vi "DataLogging_timing_test.vi"() -> ()   [LabVIEW 2018]
uses:
  Target Logging Cluster.ctl
  Logging Data Cluster.ctl
  Target Logging Control Signals.ctl
  Target Logging Sensors.ctl
  Sensor Data.ctl
  <vilib>/Platform/TimedLoop/XDataNode/timing_clust.ctl
  <vilib>/Platform/TimedLoop/XDataNode/nitl_modes.ctl
  <vilib>/Platform/TimedLoop/XDataNode/wakeup.ctl
  <vilib>/Analysis/baseanly.llb/Mean (DBL).vi
  <vilib>/platform/TimedLoop/XDataNode/XDataNode.xnode
  <vilib>/Platform/TimedLoop/XDataNode/XDNodeRunTimeDep.lvlib
  <vilib>/Analysis/NI_AALBase.lvlib
panel:
  out "mean (microseconds)":dbl format="%0.2f"
  out "Loop Duration Chart":i64(graph)
  in  "stop":bool
  out "Elapsed Time (ms)":u32
  out "Data Logging Error":errorcluster
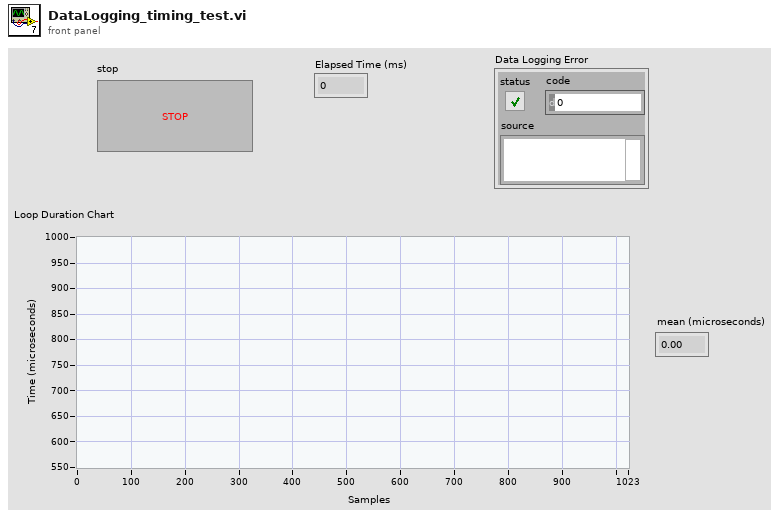
[diagram p1: front panel]
types:
  T1 = typedef "Target Logging Cluster.ctl" = cluster{"Valid for Logging?":bool, "Data":T2}
  T2 = typedef "Logging Data Cluster.ctl" = cluster{"Control Signals":T3, "Target Sensors":T4}
  T3 = typedef "Target Logging Control Signals.ctl" = cluster{"Phi":dbl, "Gait %":dbl, "ILC Desired Ankle Angle":dbl, "Desired Motor Current":dbl, "Transmission Ratio":dbl, "Passive Torque Estimate":dbl, "Torque Reference":dbl, "Left HS?":bool, "Left HS State":u32, "Right HS?":bool, "Right HS State":u32, "dGRF L":dbl, "dGRF R":dbl, "GRF L (filt) ":dbl, "GRF R (filt)":dbl}
  T4 = typedef "Target Logging Sensors.ctl" = cluster{"Sensors":T5}
  T5 = typedef "Sensor Data.ctl" = cluster{"Motor Current":dbl, "Motor Velocity":dbl, "Ankle Encoder Angle":dbl, "GRF L":dbl, "GRF R":dbl, "Index pulse?":bool, "Roll":dbl, "Pitch":dbl, "Yaw":dbl, "Thigh Angle":dbl}
  T6 = typedef "XDNodeRunTimeDep.lvlib/timing_clust.ctl" = cluster{"Expected End [f-1]":u64, "Actual End [f-1]":u64, "Finished Late? [f-1]":bool, "Expected End [i-1]":u64, "Actual End [i-1]":u64, "Finished Late? [i-1]":bool, "Expected Start [i]":u64, "Actual Start [i]":u64, "Expected Start [f]":u64, "Actual Start [f]":u64, "Source Name":string, "Structure Name":string, "Period":i64, "Deadline":i64, "Offset":i64, "Start":i64, "Priority":i32, "Timeout":i32, "Mode":T7, "Wakeup Reason":T8, "Error":errorcluster, "Source Type":string, "Secondary Source Type":string, "Global End Time":u64, "Global Start Time":u64, "Frame Duration":u64, "Iteration Duration":u64, "Assigned CPU":i32, "I/O Scan Engine Mode":u32}
  T7 = typedef "XDNodeRunTimeDep.lvlib/nitl_modes.ctl" = enum32{"No Change", "Process missed periods, maintain original phase", "Discard missed periods, maintain original phase", "Process missed periods, ignore original phase", "Discard missed periods, ignore original phase"}
  T8 = typedef "XDNodeRunTimeDep.lvlib/wakeup.ctl" = enum32{"Normal", "Aborted", "Asynchronous wakeup", "Timing source error", "Timed loop error", "Timeout"}
  T9 = typedef "Target Lossy Data.ctl" = cluster{"Active Controller":bool, "Log Trigger":bool, "Sensors":T5, "Motor Command":dbl, "Phase Variable":dbl, "Left HS State":u32, "Left Heel Strike Pulse":bool, "Gait %":dbl, "Torque Reference":dbl, "Passive Torque":dbl, "F_th":dbl, "dF_th":dbl, "d_GRF L":dbl, "GRF L":dbl, "Transmission Ratio":dbl, "Desired Ankle Traj.":dbl, "Right HS State":u32, "Right Heel Strike Pulse":bool, "d_GRF R":dbl, "GRF R":dbl}
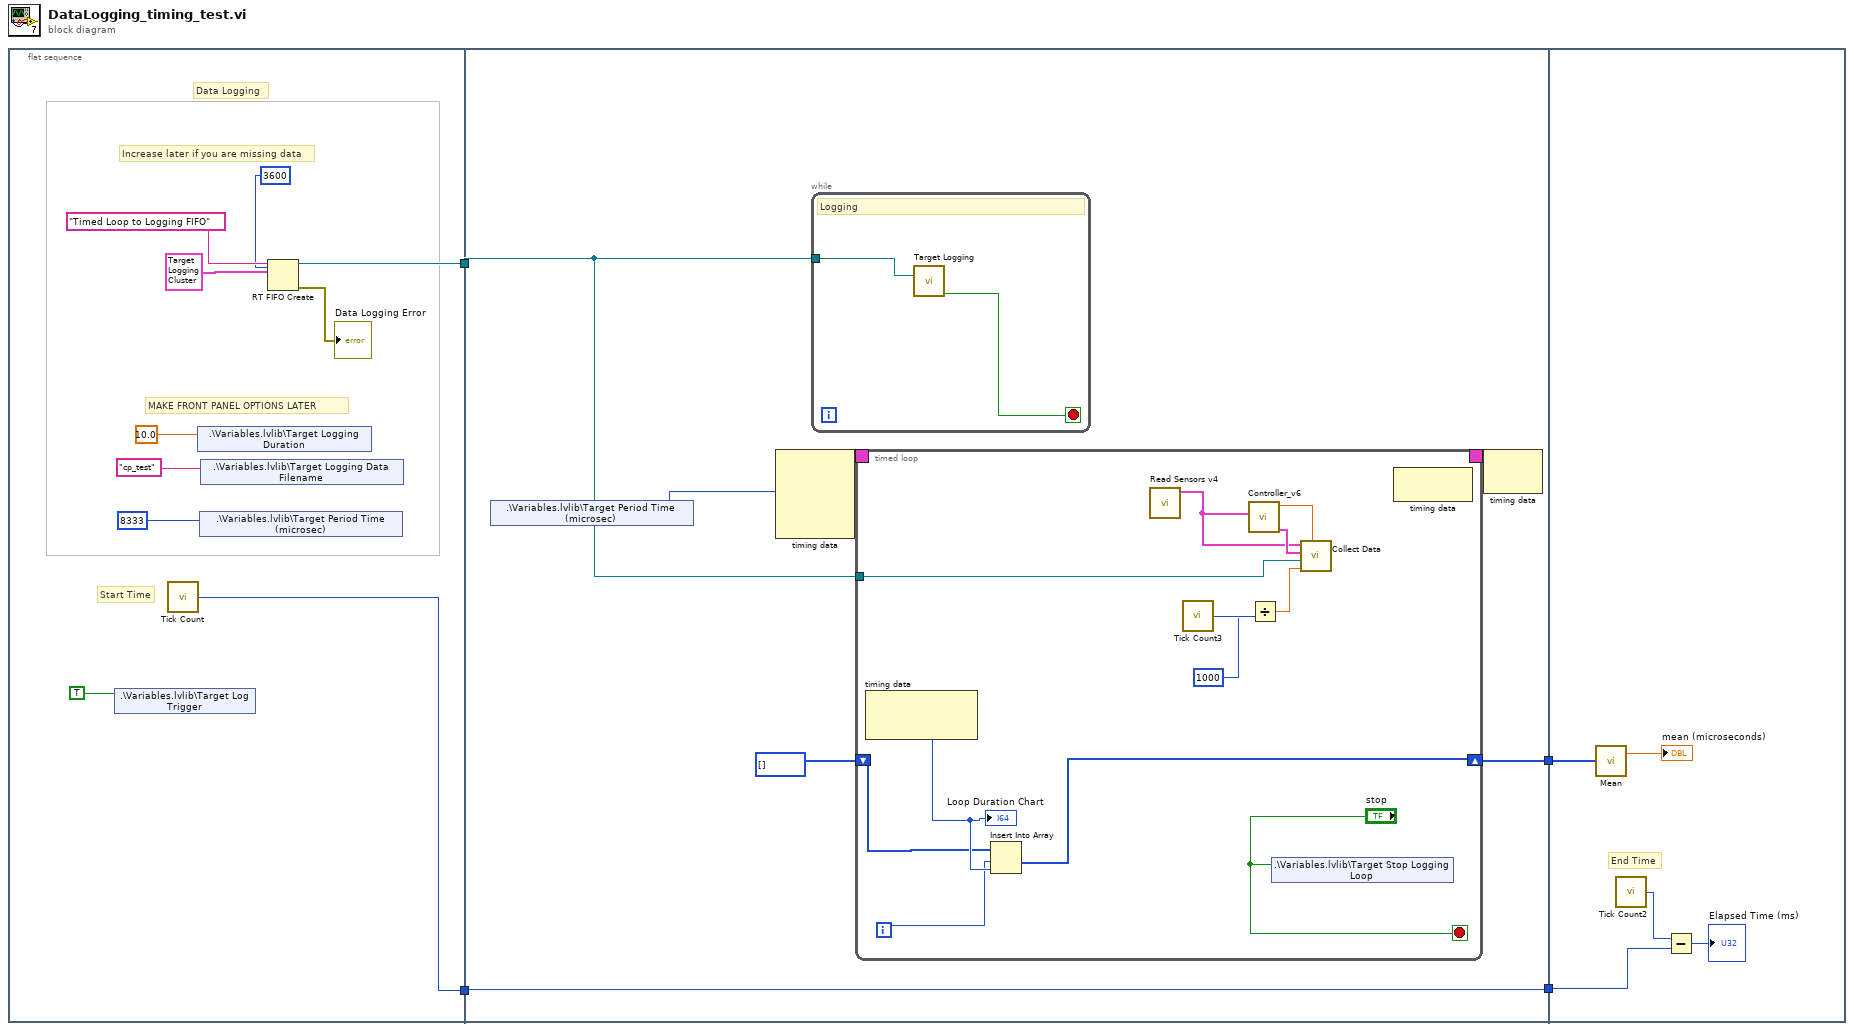
[diagram p0: block diagram]
diagram:
  n1 = flat-sequence {
    tunnel: [w7] -> w4
    tunnel: [w6] -> w2
    tunnel: w4 -> [w20]
    tunnel: [w21] -> w3
    tunnel: w2 -> [w21]
    tunnel: [w15] -> w1
    tunnel: w3 -> [w46]
    tunnel: w1 -> [w44]
    frame #0 {
      # "Start Time"
      # "MAKE FRONT PANEL OPTIONS LATER"
      # "Data Logging"
      # "Increase later if you are missing data"
      n2 = shared-variable ".\\Variables.lvlib\\Target Log Trigger"(TRUE) -> ()  [unwired: 1 in, 1 out]
      n3 = call "Tick Count"() -> ("Tick Count(mSec)"=w6:u32)
      n4 = shared-variable ".\\Variables.lvlib\\Target Logging Duration"(10.0) -> ()  [unwired: 1 in, 1 out]
      n5 = shared-variable ".\\Variables.lvlib\\Target Period Time (microsec)"(8333) -> ()  [unwired: 1 in, 1 out]
      n6 = shared-variable ".\\Variables.lvlib\\Target Logging Data Filename"("cp_test" ("Target Logging Data Filename")) -> ()  [unwired: 1 in, 1 out]
      n7 = RT FIFO Create(0:"Timed Loop to Logging FIFO" ("name (unnamed)"), 1:T1 {"Valid for Logging?"=FALSE, "Data"={"Control Signals"={"Phi"=0.0, "Gait %"=0.0, "ILC Desired Ankle Angle"=0.0, "Desired Motor Current"=0.0, "Transmission Ratio"=0.0, "Passive Torque Estimate"=0.0, "Torque Reference"=0.0, "Left HS?"=FALSE, "Left HS State"=0, "Right HS?"=FALSE, "Right HS State"=0, "dGRF L"=0.0, "dGRF R"=0.0, "GRF L (filt) "=0.0, "GRF R (filt)"=0.0}, "Target Sensors"={"Sensors"={"Motor Current"=0.0, "Motor Velocity"=0.0, "Ankle Encoder Angle"=0.0, "GRF L"=0.0, "GRF R"=0.0, "Index pulse?"=FALSE, "Roll"=0.0, "Pitch"=0.0, "Yaw"=0.0, "Thigh Angle"=0.0}}}} ("Logging Cluster"), 4:u32 3600 ("size (10)")) -> (8:w7:refnum<k33>, 11:→"Data Logging Error":errorcluster)  [unwired: 5 in, 1 out]
    }
    frame #1 {
      n8 = shared-variable ".\\Variables.lvlib\\Target Period Time (microsec)"() -> (w17:u16)  [unwired: 1 in, 1 out]
      n9 = node-c288(w17) -> (w19:T6)  [unwired: 3 in]
      n10 = while {
        tunnel: w20 -> [w41]
        stop <- w42 stop-if-true
        # "Logging"
        n11 = call "Target Logging.vi"("rt fifo"=w41) -> ("Stop Loop"=w42:bool)  [unwired: 10 in]
      }
      n12 = timed-loop {
        timing: w19 -> [_]
        timing-out: [_] -> w18
        tunnel: w20 -> [w33]
        shift-right: [w23] -> w15
        shift-left: i64[] [] -> [w24]
        i -> [w25]
        stop <- "stop" stop-if-true
        n13 = node-c288() -> (w26:i64)  [unwired: 1 in, 1 out]
        "Loop Duration Chart" <- w26
        n14 = Insert Into Array(array=w24, index=w25, new element=w26) -> (w23:i64[])
        n15 = call "Read Sensors v4.vi"() -> ("Sensors"=w27:T5)  [unwired: 10 in, 1 out]
        n16 = call "Tick Count3"() -> ("Tick Count(mSec)"=w32:u32)
        n17 = call "Controller_v6.vi"("Sensors"=w27) -> ("To Target Lossy Data"=w28:T9, "Motor Command"=w29:dbl)  [unwired: 9 in]
        n18 = Divide(x=w32, y=u32 1000) -> (x/y=w30:dbl)
        n19 = shared-variable ".\\Variables.lvlib\\Target Stop Logging Loop"("stop") -> ()  [unwired: 1 in, 1 out]
        n20 = call "Collect Data.vi"("Motor Command"=w29, "Current Time (s)"=w30, "rt fifo"=w33, "Target Lossy Data"=w28, "Sensors"=w27) -> ()  [unwired: 7 in]
        n21 = node-c288() -> ()  [unwired: 1 in, 1 out]
      }
      n22 = node-c288(w18) -> ()  [unwired: 1 out]
    }
    frame #2 {
      # "End Time"
      n23 = call-poly <vilib>:"Mean.vi"("X"=w44) -> ("mean"=→"mean (microseconds)":dbl)  [unwired: 1 out]
      n24 = call "Tick Count2"() -> ("Tick Count(mSec)"=w47:u32)
      n25 = Subtract(x=w47, y=w46) -> (x-y=→"Elapsed Time (ms)":u32)
    }
  }
